vi "controlVisibility4Ch.vi"(7 "device type [AB1004]":T2=1004 items=["any"=0, "AB1002"=1002, "AB1004"=1004], 9 "ref controls":T1, 10 "connection state":T3) -> ()   [LabVIEW 2015]
doc: "Sets the visibility of control inputs on front panel at \"Tausand AB1000 Acquisition Example.vi\", depending on the current connection state."
uses:
  <instrlib>/Tausand AB1000/Examples/sub vi/connectionState.ctl
  <instrlib>/Tausand AB1000/Public/Controls/deviceTypeRing.ctl
  <instrlib>/Tausand AB1000/Tausand AB1000.lvlib
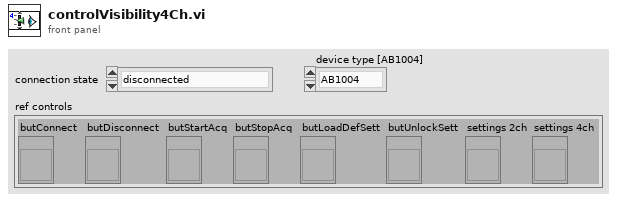
[diagram p1: front panel]
types:
  T1 = cluster{"butConnect":refnum<vi>, "butDisconnect":refnum<vi>, "butStartAcq":refnum<vi>, "butStopAcq":refnum<vi>, "butLoadDefSett":refnum<vi>, "butUnlockSett":refnum<vi>, "settings 2ch":refnum<vi>, "settings 4ch":refnum<vi>}
  T2 = typedef "Tausand AB1000.lvlib/deviceTypeRing.ctl" = u16
  T3 = typedef "connectionState.ctl" = enum16{"disconnected", "connected", "acquiring data", "connection error", "acquisition error"}
  T4 = enum8{"Enabled", "Disabled", "Disabled and Grayed Out"}
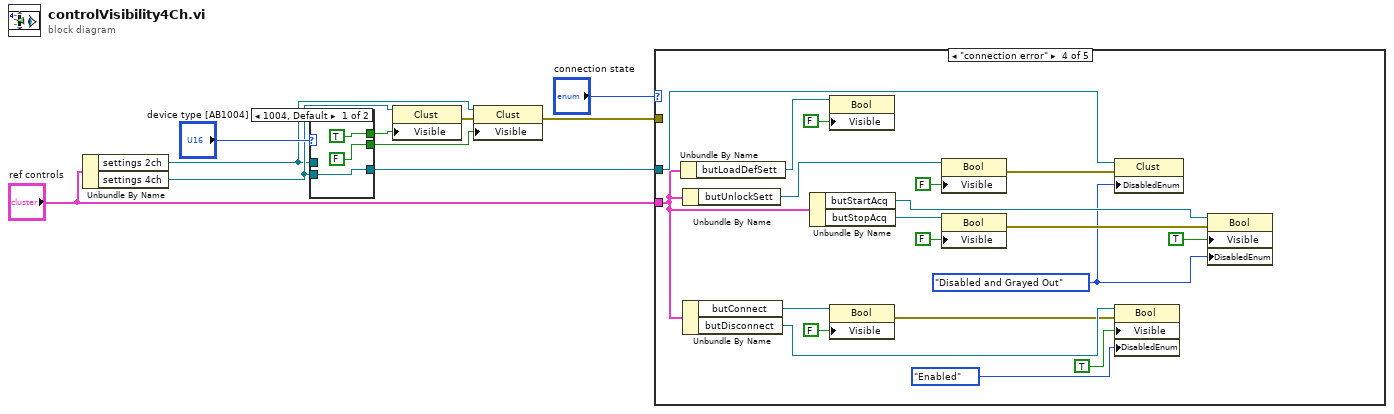
[diagram p0: block diagram]
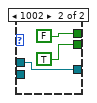
[diagram p2: hidden frame]
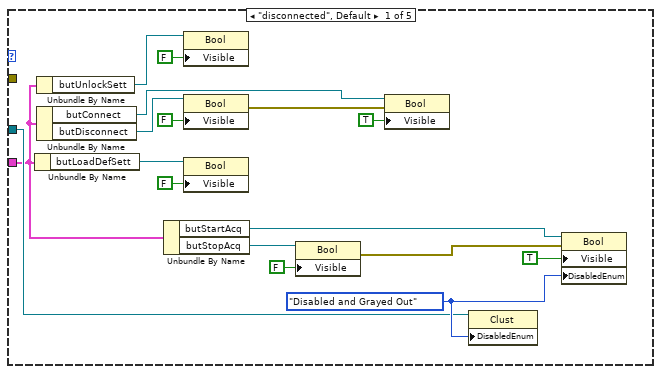
[diagram p3: hidden frame]
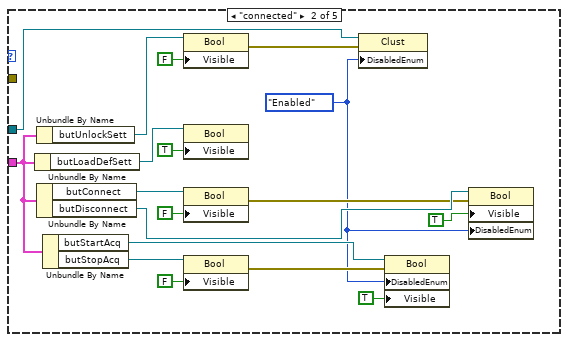
[diagram p4: hidden frame]
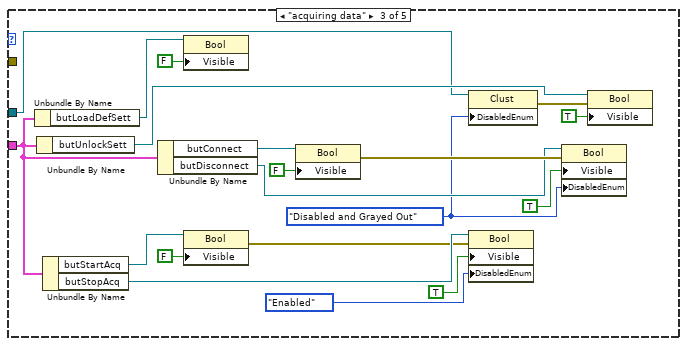
[diagram p5: hidden frame]
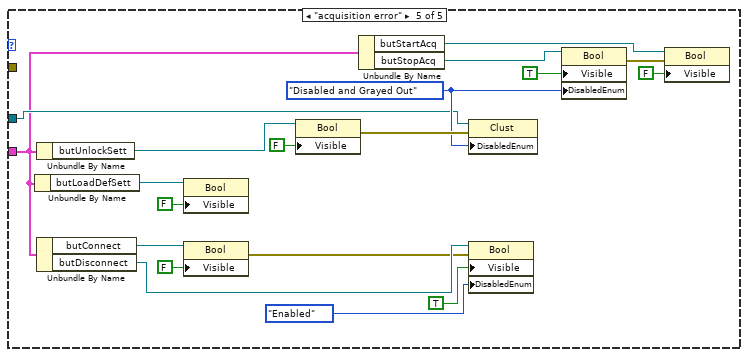
[diagram p6: hidden frame]
diagram:
  n1 = Unbundle By Name("ref controls") -> ("settings 2ch"=w3:refnum<vi>, "settings 4ch"=w4:refnum<vi>)
  n2 = case shown="1004, Default" "device type [AB1004]" {
    tunnel: [FALSE TRUE] -> w8
    tunnel: [TRUE FALSE] -> w7
    tunnel: [w11 w14] -> w2
    tunnel: w4 -> [w11 _]
    tunnel: w3 -> [_ w14]
    frame 1004, Default {
    }
    frame 1002 {
    }
  }
  n3 = property class="Clust"(reference=w4, "Visible"=w7) -> (error out=w6:errorcluster)  [unwired: 1 in, 1 out]
  n4 = property class="Clust"(reference=w3, error in=w6, "Visible"=w8) -> (error out=w5:errorcluster)  [unwired: 1 out]
  n5 = case shown="\"connection error\"" "connection state" {
    tunnel: "ref controls" -> [w17 w34 w54 w71 w90]
    tunnel: w5 -> [_ _ _ _ _]
    tunnel: w2 -> [w20 w37 w55 w74 w93]
    frame "disconnected", Default {
      w26 = T4."Disabled and Grayed Out" ("Disabled")
      n6 = Unbundle By Name(w17) -> ("butLoadDefSett"=w19:refnum<vi>)
      n7 = Unbundle By Name(w17) -> ("butUnlockSett"=w28:refnum<vi>)
      n8 = Unbundle By Name(w17) -> ("butConnect"=w24:refnum<vi>, "butDisconnect"=w23:refnum<vi>)
      n9 = Unbundle By Name(w17) -> ("butStartAcq"=w22:refnum<vi>, "butStopAcq"=w21:refnum<vi>)
      n10 = property class="Bool"(reference=w28, "Visible"=FALSE) -> ()  [unwired: 1 in, 2 out]
      n11 = property class="Bool"(reference=w23, "Visible"=FALSE) -> (error out=w25:errorcluster)  [unwired: 1 in, 1 out]
      n12 = property class="Bool"(reference=w19, "Visible"=FALSE) -> ()  [unwired: 1 in, 2 out]
      n13 = property class="Bool"(reference=w21, "Visible"=FALSE) -> (error out=w27:errorcluster)  [unwired: 1 in, 1 out]
      n14 = property class="Bool"(reference=w24, error in=w25, "Visible"=TRUE) -> ()  [unwired: 2 out]
      n15 = property class="Clust"(reference=w20, "DisabledEnum"=w26) -> ()  [unwired: 1 in, 2 out]
      n16 = property class="Bool"(reference=w22, error in=w27, "Visible"=TRUE, "DisabledEnum"=w26) -> ()  [unwired: 2 out]
    }
    frame "connected" {
      w38 = T4."Enabled" ("Disabled")
      n17 = Unbundle By Name(w34) -> ("butLoadDefSett"=w36:refnum<vi>)
      n18 = Unbundle By Name(w34) -> ("butUnlockSett"=w40:refnum<vi>)
      n19 = Unbundle By Name(w34) -> ("butConnect"=w51:refnum<vi>, "butDisconnect"=w47:refnum<vi>)
      n20 = Unbundle By Name(w34) -> ("butStartAcq"=w48:refnum<vi>, "butStopAcq"=w45:refnum<vi>)
      n21 = property class="Bool"(reference=w40, "Visible"=FALSE) -> (error out=w39:errorcluster)  [unwired: 1 in, 1 out]
      n22 = property class="Bool"(reference=w36, "Visible"=TRUE) -> ()  [unwired: 1 in, 2 out]
      n23 = property class="Bool"(reference=w51, "Visible"=FALSE) -> (error out=w46:errorcluster)  [unwired: 1 in, 1 out]
      n24 = property class="Bool"(reference=w45, "Visible"=FALSE) -> (error out=w42:errorcluster)  [unwired: 1 in, 1 out]
      n25 = property class="Clust"(reference=w37, error in=w39, "DisabledEnum"=w38) -> ()  [unwired: 2 out]
      n26 = property class="Bool"(reference=w48, error in=w42, "DisabledEnum"=w38, "Visible"=TRUE) -> ()  [unwired: 2 out]
      n27 = property class="Bool"(reference=w47, error in=w46, "Visible"=TRUE, "DisabledEnum"=w38) -> ()  [unwired: 2 out]
    }
    frame "acquiring data" {
      w59 = T4."Disabled and Grayed Out" ("Disabled")
      n28 = Unbundle By Name(w54) -> ("butLoadDefSett"=w52:refnum<vi>)
      n29 = Unbundle By Name(w54) -> ("butUnlockSett"=w57:refnum<vi>)
      n30 = Unbundle By Name(w54) -> ("butStartAcq"=w70:refnum<vi>, "butStopAcq"=w69:refnum<vi>)
      n31 = Unbundle By Name(w54) -> ("butConnect"=w61:refnum<vi>, "butDisconnect"=w60:refnum<vi>)
      n32 = property class="Bool"(reference=w52, "Visible"=FALSE) -> ()  [unwired: 1 in, 2 out]
      n33 = property class="Bool"(reference=w70, "Visible"=FALSE) -> (error out=w66:errorcluster)  [unwired: 1 in, 1 out]
      n34 = property class="Bool"(reference=w61, "Visible"=FALSE) -> (error out=w62:errorcluster)  [unwired: 1 in, 1 out]
      n35 = property class="Clust"(reference=w55, "DisabledEnum"=w59) -> (error out=w56:errorcluster)  [unwired: 1 in, 1 out]
      n36 = property class="Bool"(reference=w69, error in=w66, "Visible"=TRUE, "DisabledEnum"=T4."Enabled" ("Disabled")) -> ()  [unwired: 2 out]
      n37 = property class="Bool"(reference=w60, error in=w62, "Visible"=TRUE, "DisabledEnum"=w59) -> ()  [unwired: 2 out]
      n38 = property class="Bool"(reference=w57, error in=w56, "Visible"=TRUE) -> ()  [unwired: 2 out]
    }
    frame "connection error" {
      w75 = T4."Disabled and Grayed Out" ("Disabled")
      n39 = Unbundle By Name(w71) -> ("butLoadDefSett"=w73:refnum<vi>)
      n40 = Unbundle By Name(w71) -> ("butUnlockSett"=w79:refnum<vi>)
      n41 = Unbundle By Name(w71) -> ("butConnect"=w89:refnum<vi>, "butDisconnect"=w85:refnum<vi>)
      n42 = Unbundle By Name(w71) -> ("butStartAcq"=w86:refnum<vi>, "butStopAcq"=w83:refnum<vi>)
      n43 = property class="Bool"(reference=w73, "Visible"=FALSE) -> ()  [unwired: 1 in, 2 out]
      n44 = property class="Bool"(reference=w89, "Visible"=FALSE) -> (error out=w84:errorcluster)  [unwired: 1 in, 1 out]
      n45 = property class="Bool"(reference=w79, "Visible"=FALSE) -> (error out=w78:errorcluster)  [unwired: 1 in, 1 out]
      n46 = property class="Bool"(reference=w83, "Visible"=FALSE) -> (error out=w81:errorcluster)  [unwired: 1 in, 1 out]
      n47 = property class="Clust"(reference=w74, error in=w78, "DisabledEnum"=w75) -> ()  [unwired: 2 out]
      n48 = property class="Bool"(reference=w85, error in=w84, "Visible"=TRUE, "DisabledEnum"=T4."Enabled" ("Disabled")) -> ()  [unwired: 2 out]
      n49 = property class="Bool"(reference=w86, error in=w81, "Visible"=TRUE, "DisabledEnum"=w75) -> ()  [unwired: 2 out]
    }
    frame "acquisition error" {
      w94 = T4."Disabled and Grayed Out" ("Disabled")
      n50 = Unbundle By Name(w90) -> ("butLoadDefSett"=w92:refnum<vi>)
      n51 = Unbundle By Name(w90) -> ("butUnlockSett"=w98:refnum<vi>)
      n52 = Unbundle By Name(w90) -> ("butConnect"=w108:refnum<vi>, "butDisconnect"=w104:refnum<vi>)
      n53 = property class="Bool"(reference=w92, "Visible"=FALSE) -> ()  [unwired: 1 in, 2 out]
      n54 = property class="Bool"(reference=w108, "Visible"=FALSE) -> (error out=w103:errorcluster)  [unwired: 1 in, 1 out]
      n55 = property class="Bool"(reference=w98, "Visible"=FALSE) -> (error out=w97:errorcluster)  [unwired: 1 in, 1 out]
      n56 = Unbundle By Name(w90) -> ("butStartAcq"=w105:refnum<vi>, "butStopAcq"=w102:refnum<vi>)
      n57 = property class="Clust"(reference=w93, error in=w97, "DisabledEnum"=w94) -> ()  [unwired: 2 out]
      n58 = property class="Bool"(reference=w104, error in=w103, "Visible"=TRUE, "DisabledEnum"=T4."Enabled" ("Disabled")) -> ()  [unwired: 2 out]
      n59 = property class="Bool"(reference=w102, "Visible"=TRUE, "DisabledEnum"=w94) -> (error out=w100:errorcluster)  [unwired: 1 in, 1 out]
      n60 = property class="Bool"(reference=w105, error in=w100, "Visible"=FALSE) -> ()  [unwired: 2 out]
    }
  }
